vi "Cannon Process.vi"(0 "error in":errorcluster) -> ()   [LabVIEW 2012]
uses:
  Cannon Global Data.vi
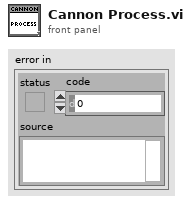
[diagram p1: front panel]
types:
  T1 = cluster{"RPM":dbl, "Trigger":bool, "Angle Axis":dbl, "Angle":dbl, "Throttle":dbl, "Slow Angle Change?":bool, "Angle Change?":bool}
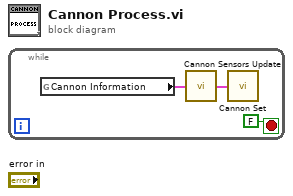
[diagram p0: block diagram]
diagram:
  n1 = while {
    stop <- FALSE stop-if-true
    n2 = global read "Cannon Global Data.vi" "Cannon Information"() -> (w3:T1)
    n3 = call "Cannon Sensors Update.vi"("Cannon Information"=w3) -> ("Cannon Information out"=w2:T1)
    n4 = call "Cannon Set.vi"("Cannon Information"=w2) -> ()
  }
